vi "SubType.vi"(7 "type":i16[](array[numeric]), 10 "Offset In":i16) -> (0 "Size":i16, 1 "subtype":i16[](array[numeric]), 2 "Offset out":i16)   [LabVIEW 2020, in "JSONtext.lvlib" / "SetMap.lvlib"]
uses:
  <vilib>/JDP Science/JSONtext/support/Set Map/SetMap.lvlib
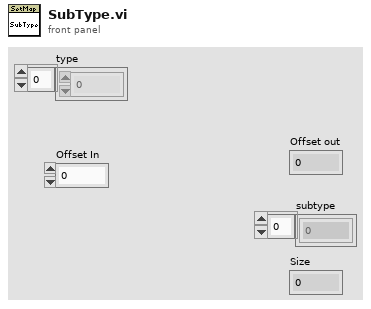
[diagram p1: front panel]
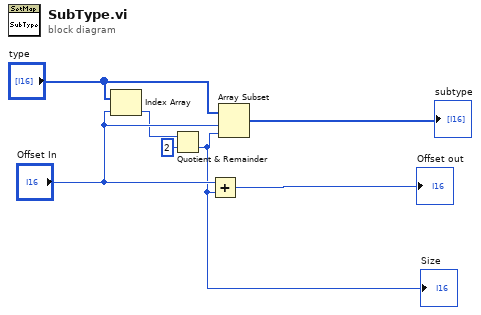
[diagram p0: block diagram]
diagram:
  n1 = Index Array(array="type", index="Offset In") -> (element=w3:i16)
  n2 = Quotient & Remainder(x=w3, y=i16 2) -> (floor(x/y)=w2:i16)  [unwired: 1 out]
  "Size" <- w2
  n3 = Add(x="Offset In", y=w2) -> (x+y=→"Offset out":i16)
  n4 = Array Subset(array="type", index="Offset In", length=w2) -> (→"subtype":i16[])
